vi "try_Create Timing Sequence.vi"() -> ()   [LabVIEW 2020]
uses:
  <vilib>/Analysis/NI_AALPro.lvlib
  <vilib>/Analysis/NI_AALBase.lvlib
  <vilib>/Analysis/Matrix/NI_Matrix.lvlib
  <vilib>/Analysis/7linalg.llb/Eigenvalue and Vectors Output Option.ctl
  <vilib>/Analysis/baseanly.llb/Real A x B.vi
  <vilib>/Analysis/7linalg.llb/Real Eigenvalues and Vectors.vi
  <vilib>/Analysis/baseanly.llb/Complex A x B.vi
  <vilib>/Analysis/Matrix/Numeric/Complex/Complex To Cartesian - CM.vi
  <vilib>/Analysis/7linalg.llb/Create Special Complex Matrix.vi
  <vilib>/Analysis/7linalg.llb/Create Special Real Matrix.vi
panel:
  out "Real Matrix R":dbl[][](array[numeric])
  in  "Expected Values":dbl[](array[numeric])
  in  "B":dbl[][](array[numeric])
  in  "Input Vector":dbl[](array[numeric])
  # "Create Timing Sequence Demo"
  # "See the block diagram."
  # "Close this VI when you are done with the demo."
  # "You do not need to save changes to this VI."
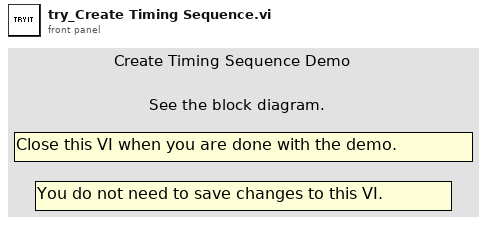
[diagram p1: front panel]
types:
  T1 = typedef "NI_AALPro.lvlib/Eigenvalue and Vectors Output Option.ctl" = i32
  T2 = typedef "NI_Matrix.lvlib/RealMatrix.ctl" = dbl[][]
  T3 = typedef "NI_Matrix.lvlib/ComplexMatrix.ctl" = cdb[][]
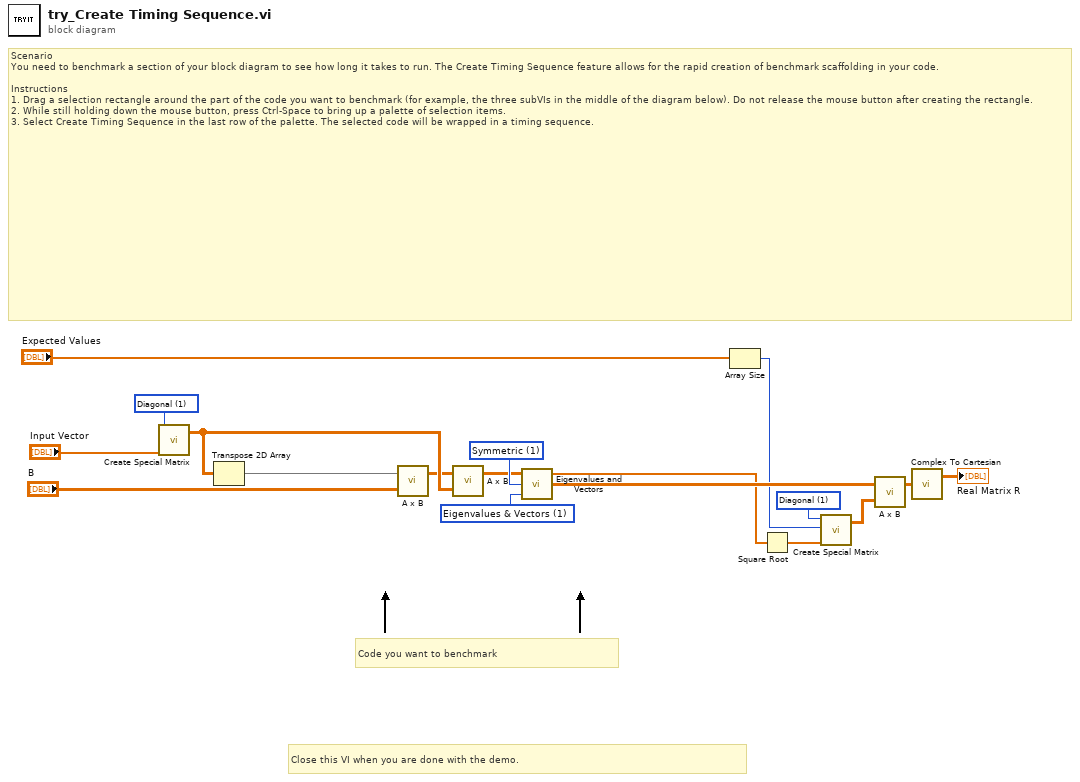
[diagram p0: block diagram]
diagram:
  w18 = 1 items=["Identity", "Diagonal", "Toeplitz", "Vandermonde", "Companion", "Hankel", "Hadamard", "Wilkinson", "Hilbert", "Inverse Hilbert", "Rosser", "Pascal"] ("matrix type")
  w6 = 1 items=["Identity", "Diagonal", "Toeplitz", "Vandermonde", "Companion", "Hankel", "Hadamard", "Wilkinson", "Hilbert", "Inverse Hilbert", "Rosser", "Pascal"] ("matrix type")
  w7 = T1 1 items=["Eigenvalues", "Eigenvalues & Vectors"] ("output option")
  w8 = 1 items=["General", "Symmetric"] ("matrix type")
  # "Close this VI when you are done with the demo."
  # "Code you want to benchmark"
  # "Scenario\nYou need to benchmark a section of your block diagram to see how long it takes to run. The Create Timing Sequence feature allows for the rapid creation of benchmark scaffolding in your code.\n\nInstructions\n1. Drag a selection rectangle around the part of the code you want to benchmark (for example, the three subVIs in the middle of the diagram below). Do not release the mouse button after creating the rectangle.\n2. While still holding down the mouse button, press Ctrl-Space to bring up a palette of selection items.\n3. Select Create Timing Sequence in the last row of the palette. The selected code will be wrapped in a timing sequence."
  n1 = call-poly <vilib>:"Create Special Matrix.vi"("matrix type"=w18, "Input Vector1"="Input Vector") -> ("Special Matrix"=w16:T2)  [unwired: 3 in, 1 out]
  n2 = Transpose 2D Array(2D array=w16) -> (transposed array=w17:T2)
  n3 = call-poly <vilib>:"A x B.vi"("B"="B", "A"=w17) -> ("A x B"=w15:T2)  [unwired: 1 out]
  n4 = call-poly <vilib>:"A x B.vi"("B"=w16, "A"=w15) -> ("A x B"=w5:T2)  [unwired: 1 out]
  n5 = call-poly <vilib>:"Eigenvalues and Vectors.vi"("output option"=w7, "matrix type"=w8, "Input Matrix"=w5) -> ("Eigenvectors"=w13:T3, "Eigenvalues"=w12:cdb[])  [unwired: 1 out]
  n6 = Array Size(array="Expected Values") -> (size(s)=w9:i32)
  n7 = Square Root(x=w12) -> (sqrt(x)=w11:cdb[])
  n8 = call-poly <vilib>:"Create Special Matrix.vi"("matrix type"=w6, "matrix size"=w9, "Input Vector1"=w11) -> ("Special Matrix"=w14:T3)  [unwired: 1 in, 2 out]
  n9 = call-poly <vilib>:"A x B.vi"("B"=w14, "A"=w13) -> ("A x B"=w10:T3)  [unwired: 1 out]
  n10 = call-poly <vilib>:"Complex To Cartesian.vi"("Complex Matrix R + Ii"=w10) -> ("Real Matrix R"=→"Real Matrix R":T2)  [unwired: 1 out]
